vi "Get Unsubscribe Data.vi"(8 "error in (no error)":errorcluster, 11 "Topic Actor Unsubscribe Command in":refnum<class "Topic Actor Unsubscribe Command.lvclass">) -> (0 "error out":errorcluster, 2 "Subscriber Name":string, 3 "Topic Actor Unsubscribe Command out":refnum<class "Topic Actor Unsubscribe Command.lvclass">)   [LabVIEW 2016, in "Stream Mediator.lvlib" / "Topic Actor Unsubscribe Command.lvclass"]
doc: "--\nCopyright © 2017 Composed SystemsI All rights reserved.\n\nAuthor: Jon McBee <jon.mcbee@composed.io>\n\nThis library is provided \"AS IS\" ,WITHOUT WARRANTIES OR\nCONDITIONS OF ANY KIND, either express or implied.\n\nComposed Systems -- composed.io\n\nStream 0.0.1.1\nJon McBee - Composed Systems\nCopyright (c) 2017, Composed Systems"
uses:
  <userlib>/Composed Systems/Stream/Mediator/Classes/Topic Actor Unsubscribe Command/Topic Actor Unsubscribe Command.lvclass
  <userlib>/Composed Systems/Stream/Mediator/Classes/Topic Actor Unsubscribe Command/Topic Actor Unsubscribe Command.lvclass/Topic Actor Unsubscribe Command.ctl
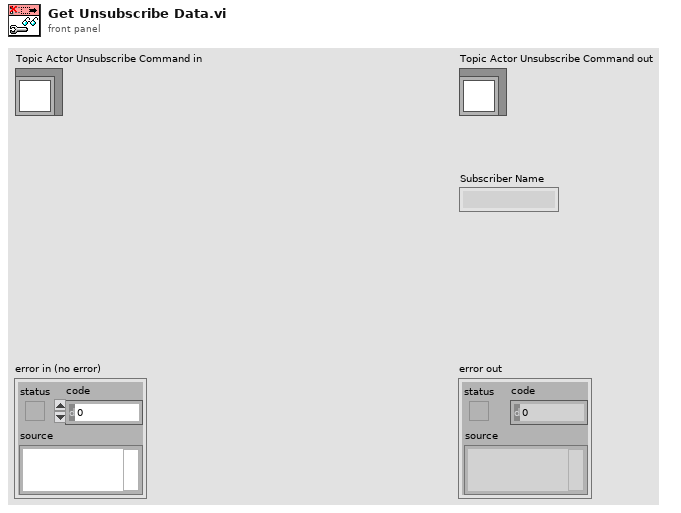
[diagram p1: front panel]
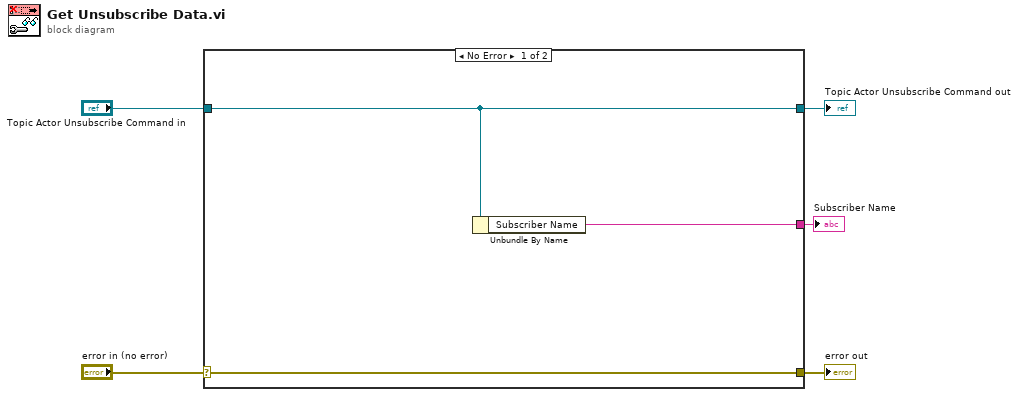
[diagram p0: block diagram]
diagram:
  n1 = case shown="No Error" "error in (no error)" {
    selector: "error in (no error)" -> [w8 w10]
    tunnel: [w8 w10] -> w4
    tunnel: [w7 w9] -> w2
    tunnel: "Topic Actor Unsubscribe Command in" -> [w7 w9]
    tunnel: [w6 _] -> w1
    frame No Error {
      n2 = Unbundle By Name(w7) -> ("Subscriber Name"=w6:string)
    }
    frame Error {
    }
  }
  "error out" <- w4
  "Topic Actor Unsubscribe Command out" <- w2
  "Subscriber Name" <- w1
